vi "调试助手.vi"() -> ()   [LabVIEW 2016]
panel:
  in  "退出":bool
  out "本机IP地址":string
  in  "端口号 2":u16=8848 caption="端口"
  in  "ledoff":bool
  in  "ledon":bool
  in  "发送按钮":bool
  in  "发送内容：":string
  out "接收数据":string
  out "错误输出":errorcluster
  out "remote address":string caption="控制器ip"
  in  "timeout ms (wait forever: -1)":i32=-1 caption="超时毫秒（一直等待:-1）"
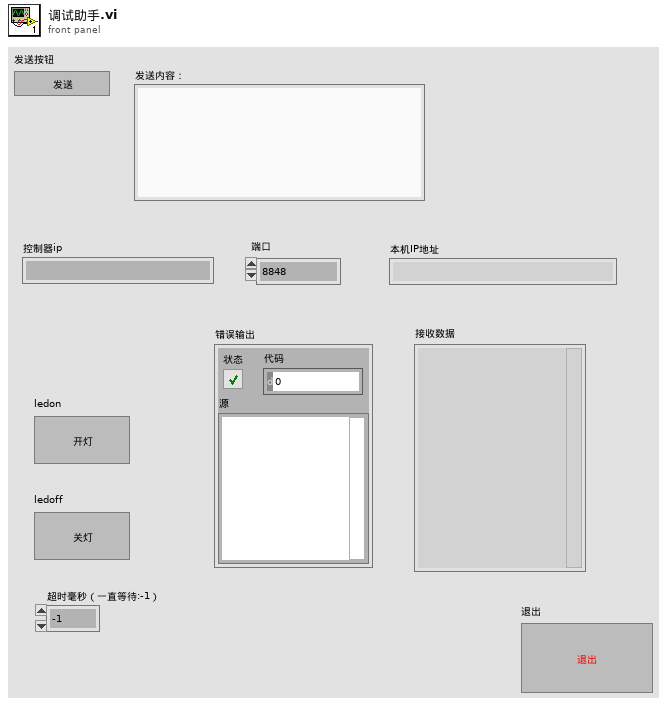
[diagram p1: front panel]
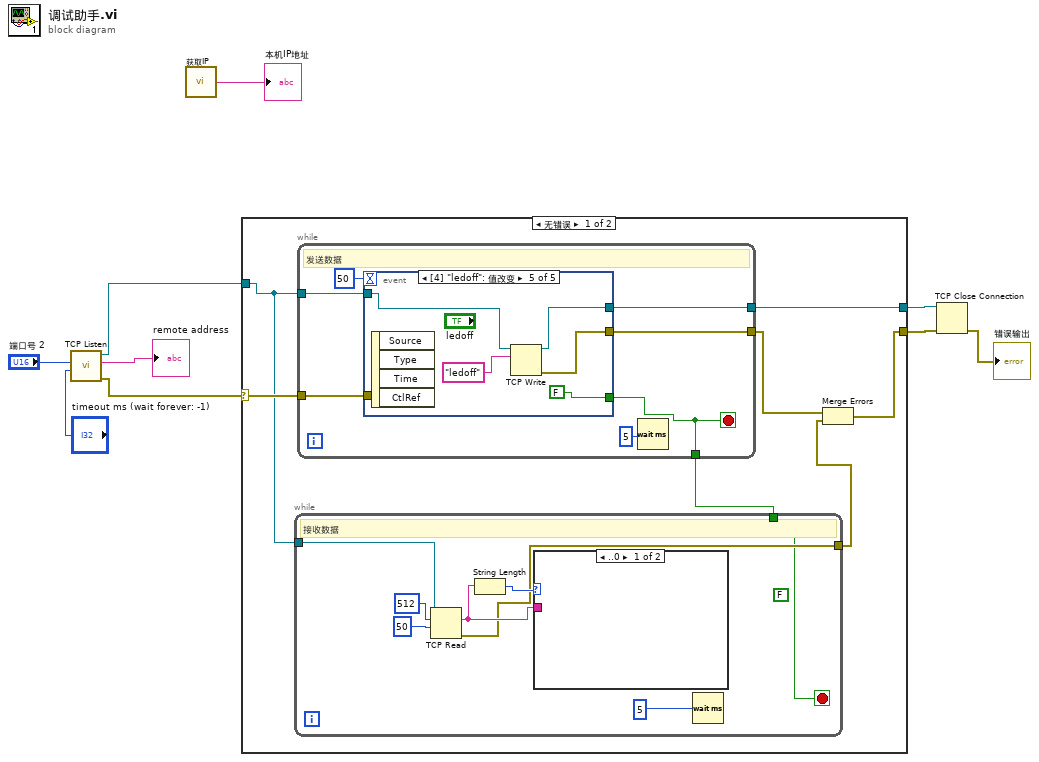
[diagram p0: block diagram]
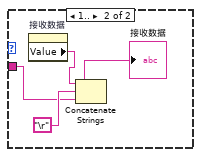
[diagram p2: hidden frame]
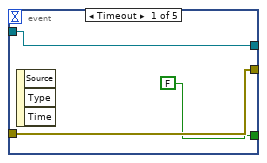
[diagram p3: hidden frame]
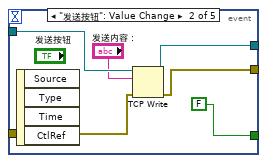
[diagram p4: hidden frame]
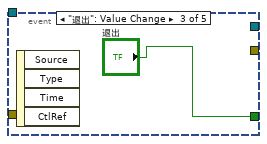
[diagram p5: hidden frame]
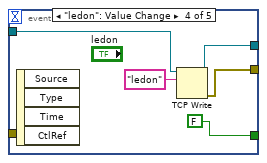
[diagram p6: hidden frame]
diagram:
  n1 = call <vilib>:"TCP Listen.vi"("timeout ms (wait forever: -1)"="timeout ms (wait forever: -1)", "port"="端口号 2") -> ("error out"=w4:errorcluster, "remote address"=→"remote address":string, "connection ID"=w5:refnum<k5>)  [unwired: 5 in, 2 out]
  n2 = call "获取IP.vi"() -> ("IP地址"=→"本机IP地址":string)  [unwired: 1 in]
  n3 = case shown="无错误" w4 {
    selector: w4 -> [w15 w56]
    tunnel: w5 -> [w14 w57]
    tunnel: [w12 w56] -> w7
    tunnel: [w16 w57] -> w8
    frame No Error {
      n4 = while {
        tunnel: w14 -> [w34]
        tunnel: [w33] -> w13
        tunnel: [w32] -> w16
        tunnel: w15 -> [w31]
        tunnel: [w29] -> w10
        stop <- w29 stop-if-true
        # "发送数据"
        n5 = event shown="[4] \"ledoff\": 值改变" {
          selector: _ -> [_ _ _ _ _]
          dyn-events: _ -> [_ _ _ _ _]
          timeout: 50 -> [_ _ _ _ _]
          tunnel: w34 -> [w38 w42 _ w50 w54]
          tunnel: [w37 w44 _ w48 w52] -> w33
          tunnel: [w38 w43 _ w47 w53] -> w32
          tunnel: w31 -> [w37 w41 _ _ _]
          tunnel: [FALSE FALSE "退出" FALSE FALSE] -> w29
          event Timeout {
            n6 = event-data() -> ()  [unwired: 1 in, 3 out]
          }
          event "发送按钮": Value Change {
            n7 = event-data() -> ()  [unwired: 1 in, 4 out]
            n8 = TCP Write(connection ID=w42, data in="发送内容：", error in (no error)=w41) -> (connection ID out=w43:refnum<k5>, error out=w44:errorcluster)  [unwired: 1 in, 1 out]
          }
          event "退出": Value Change {
            n9 = event-data() -> ()  [unwired: 1 in, 4 out]
          }
          event "ledon": Value Change {
            n10 = event-data() -> ()  [unwired: 1 in, 4 out]
            n11 = TCP Write(connection ID=w50, data in="ledon" ("数据输入")) -> (connection ID out=w47:refnum<k5>, error out=w48:errorcluster)  [unwired: 2 in, 1 out]
          }
          event "ledoff": Value Change {
            n12 = event-data() -> ()  [unwired: 1 in, 4 out]
            n13 = TCP Write(connection ID=w54, data in="ledoff" ("数据输入")) -> (connection ID out=w53:refnum<k5>, error out=w52:errorcluster)  [unwired: 2 in, 1 out]
          }
        }
        n14 = Wait (ms)(milliseconds to wait=u32 5 ("等待时间（毫秒）")) -> ()  [unwired: 1 out]
      }
      n15 = while {
        tunnel: w14 -> [w21]
        tunnel: [w18] -> w11
        tunnel: w10 -> [w17]
        stop <- w17 stop-if-true
        (unwired) FALSE
        # "接收数据"
        n16 = TCP Read(connection ID=w21, bytes to read=512, 9:50) -> (data out=w19:string, error out=w18:errorcluster)  [unwired: 2 in, 1 out]
        n17 = String Length(string=w19) -> (length=w20:i32)
        n18 = case shown="..0" w20 {
          tunnel: w19 -> [_ w25]
          frame ..0 {
          }
          frame 1.. {
            n19 = property on="接收数据" class="Str"() -> ("Value"=w27:string)  [unwired: 2 in, 2 out]
            n20 = Concatenate Strings(w27, "\r", w25) -> (→"接收数据":string)
          }
        }
        n21 = Wait (ms)(milliseconds to wait=u32 5 ("等待时间（毫秒）")) -> ()  [unwired: 1 out]
      }
      n22 = Merge Errors(w13, w11) -> (w12:errorcluster)
    }
    frame Error {
    }
  }
  n23 = TCP Close Connection(connection ID=w8, error in (no error)=w7) -> (error out=→"错误输出":errorcluster)  [unwired: 1 in, 1 out]
